vi "Read Inputs from system.vi"(8 "error in":errorcluster, 11 "My Awesome Control Modules runtime in":refnum<class "My Awesome Control Modules runtime.lvclass">) -> (0 "error out":errorcluster, 2 "Inputs from system":T1, 3 "My Awesome Control Modules runtime out":refnum<class "My Awesome Control Modules runtime.lvclass">)   [LabVIEW 2013, in "My Awesome Control Modules runtime.lvclass"]
uses:
  My Awesome Control Modules runtime.lvclass
  configuration/input data indices.ctl
  configuration/My Awesome Control Modules configuration.lvclass
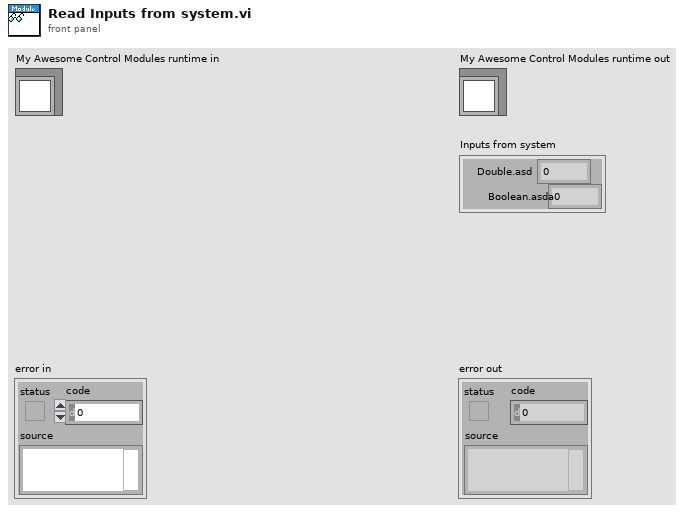
[diagram p1: front panel]
types:
  T1 = typedef "My Awesome Control Modules configuration.lvclass/input data indices.ctl" = cluster{"Double.asd":i32, "Boolean.asda":i32}
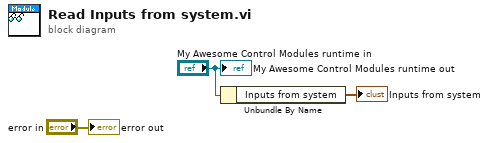
[diagram p0: block diagram]
diagram:
  n1 = Unbundle By Name("My Awesome Control Modules runtime in") -> ("Inputs from system"=→"Inputs from system":T1)
  "error out" <- "error in"
  "My Awesome Control Modules runtime out" <- "My Awesome Control Modules runtime in"
